vi "WS1050 OFFSET CAL.vi"(8 "error in":errorcluster, 10 "OFFSET CAL":bool=TRUE) -> (0 "error out":errorcluster)   [LabVIEW 2012]
uses:
  WS_VCAP Driver 029/Source/WSVCAP Shell/Type Defs/WSVCAP SHL I2C DUT Mask Mode Enum.ctl
panel:
  out "AD7747 Values":string[][](table)
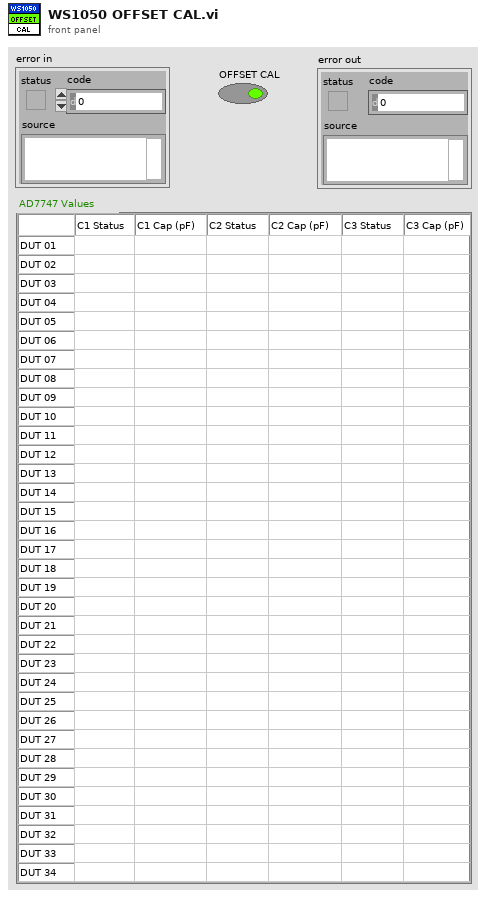
[diagram p1: front panel]
types:
  T1 = typedef "WSVCAP SHL I2C DUT Mask Mode Enum.ctl" = enum16{"Custom", "C1", "C2", "C3", "All"}
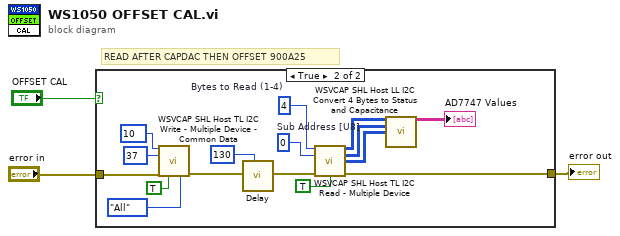
[diagram p0: block diagram]
diagram:
  # "READ AFTER CAPDAC THEN OFFSET 900A25"
  n1 = case shown="True" "OFFSET CAL" {
    tunnel: "error in" -> [w4 w20]
    tunnel: [w4 w14] -> w3
    frame False {
    }
    frame True {
      w18 = u8 4  # Bytes to Read (1-4)
      w19 = u8 0  # Sub Address [U8]
      n2 = call "WSVCAP SHL Host TL I2C Write - Multiple Device - Common Data.vi"("Sub Address"=u8 10, "Data Out [U8]"=u8 37 ("Sub Address"), "error in"=w20, "Log (T)"=TRUE, "DUT Mask Mode (All)"=WSVCAP_SHL_I2C_DUT_Mask_Mode_Enum."All") -> ("error out"=w7:errorcluster)  [unwired: 10 in]
      n3 = call "Delay.vi"("milliseconds to wait"=u32 130, "error in (no error)"=w7) -> ("error out"=w6:errorcluster)  [unwired: 9 in]
      n4 = call "WSVCAP SHL Host TL I2C Read - Multiple Device.vi"("Bytes to Read (1-4)"=w18, "Sub Address [U8]"=w19, "error in"=w6, "Log (T)"=TRUE) -> ("C1:1-36 Read Data [U8]"=w17:u8[][], "C2:1-36 Read Data [U8]"=w16:u8[][], "C3:1-36 Read Data [U8]"=w15:u8[][], "error out"=w14:errorcluster)  [unwired: 8 in]
      n5 = call "WSVCAP SHL Host LL I2C Convert 4 Bytes to Status and Capacitance.vi"("C1:1-36 Read Data [U8]"=w17, "C2_1-36 Read Data [U8]"=w16, "C3_1-36 Read Data [U8]"=w15) -> ("AD7747 Values"=→"AD7747 Values":string[][])  [unwired: 12 in]
    }
  }
  "error out" <- w3
